vi "Main.vi"(8 "Error In":errorcluster, 11 "Simulate hardware?":bool) -> (0 "Error Out":errorcluster)   [LabVIEW 2017, in "Colour Wheel.lvlib"]
uses:
  Colour Wheel.lvlib
  Controls/Commands [enum].ctl
  Controls/Params.ctl
  Events/Controls/Action Refs [enum].ctl
  <vilib>/Utility/error.llb/Error Cluster From Error Code.vi
  <vilib>/ErrorRing/Error Ring.xnode
  System Control/Main controller.lvlib
  File IO/File IO.lvlib
  Events/Events.lvlib
  Thorlabs_FW102C/Thorlabs_FW102C.lvlib
panel:
  in  "Index":i32=1
  out "Connected?":bool
  out "COM Ports":string[](array[string])
  out "Test":bool=TRUE
  in  "Config":T1
  out "Config out":T1
  in  "Set state":T2
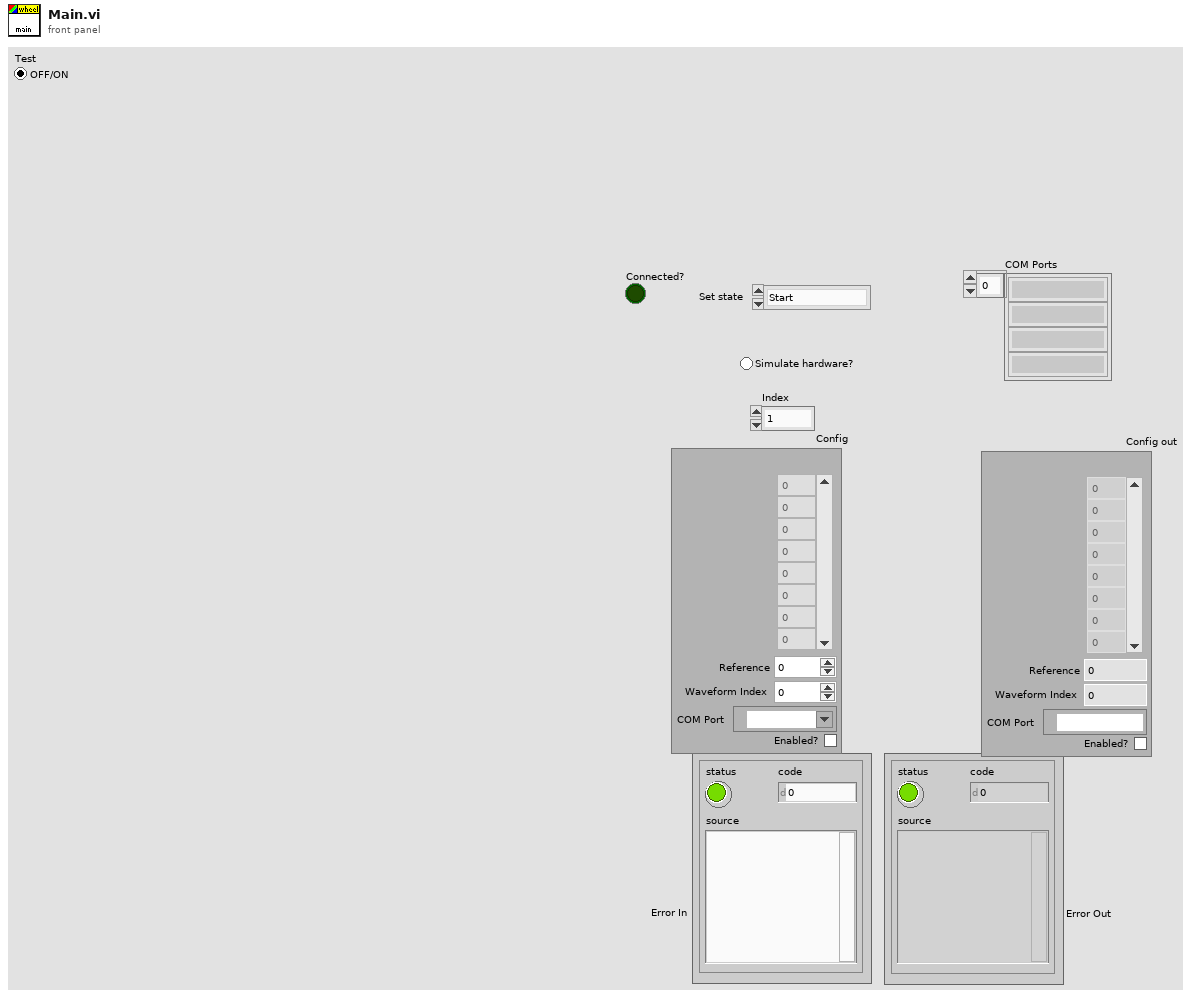
[diagram p1: front panel]
types:
  T1 = typedef "Colour Wheel.lvlib/Params.ctl" = cluster{"Reference":i32, "Colour Wheel Wavelengths":dbl[], "Waveform Index":i32, "COM Port":refnum<visa-resource-name>, "Enabled?":bool}
  T2 = typedef "Colour Wheel.lvlib/Commands [enum].ctl" = enum16{"Start", "Move", "Get position", "Stop", "Send data"}
  T3 = enum32{"Bad", "Idle", "Run top level", "Running"}
  T4 = typedef "Events.lvlib/Action Refs [enum].ctl" = enum16{"Init", "Ref", "Kill"}
  T5 = typedef "Events.lvlib/Refs [cluster].ctl" = cluster{"Exit":refnum<user-event>, "Controller":refnum<user-event>, "System Error":refnum<user-event>, "UI":refnum<user-event>, "Example Module":refnum<user-event>, "Shutter":refnum<user-event>, "Monochromator":refnum<user-event>, "DAQ":refnum<user-event>, "Scope":refnum<user-event>, "Processing":refnum<user-event>, "File IO":refnum<user-event>, "Colour wheel":refnum<user-event>}
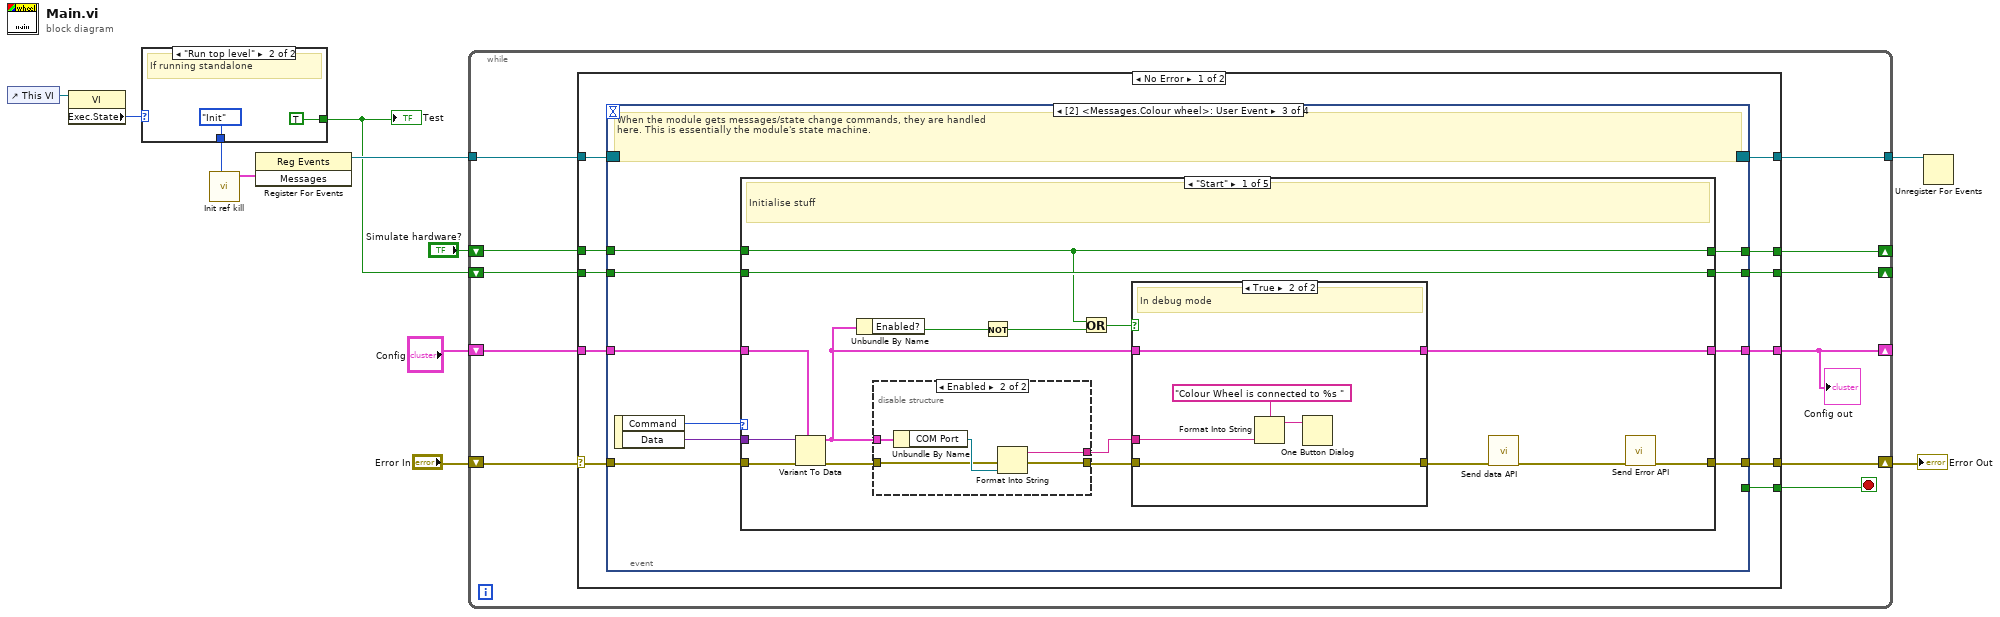
[diagram p0: block diagram]
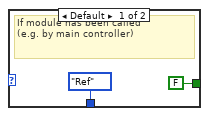
[diagram p2: hidden frame]
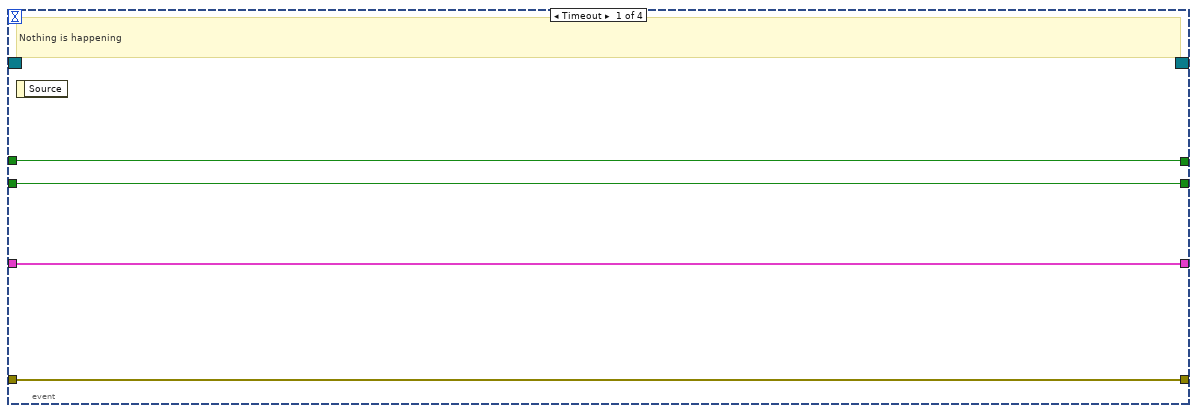
[diagram p3: hidden frame]
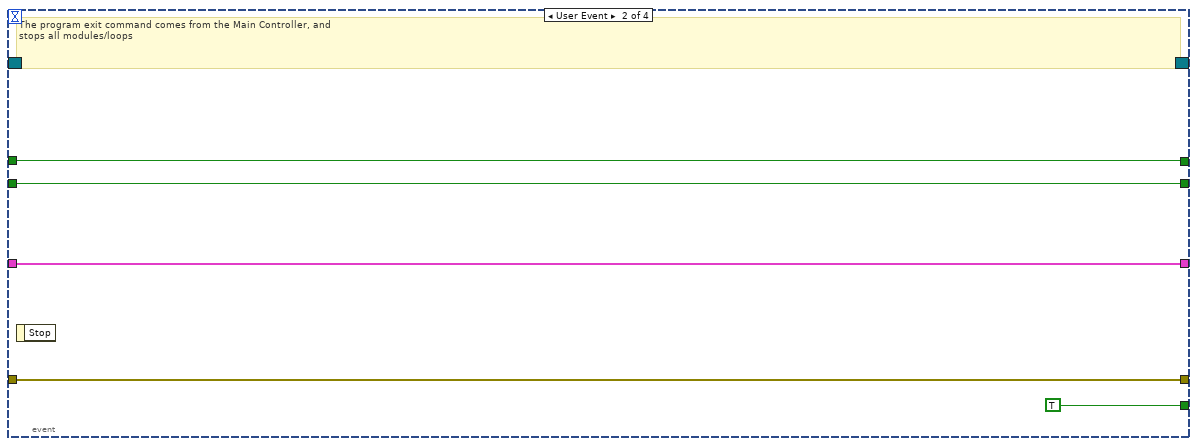
[diagram p4: hidden frame]
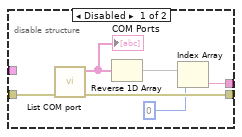
[diagram p5: hidden frame]
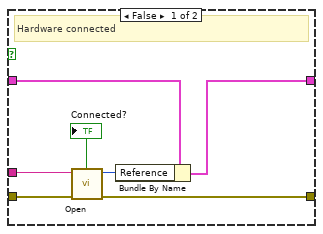
[diagram p6: hidden frame]
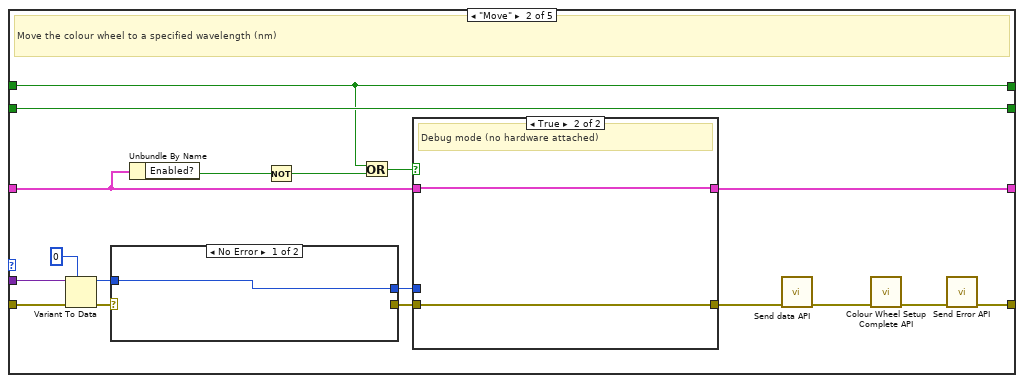
[diagram p7: hidden frame]
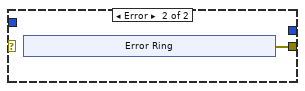
[diagram p8: hidden frame]
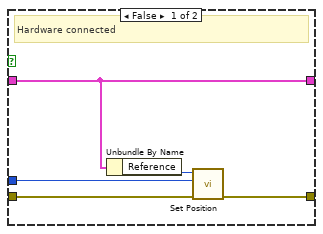
[diagram p9: hidden frame]
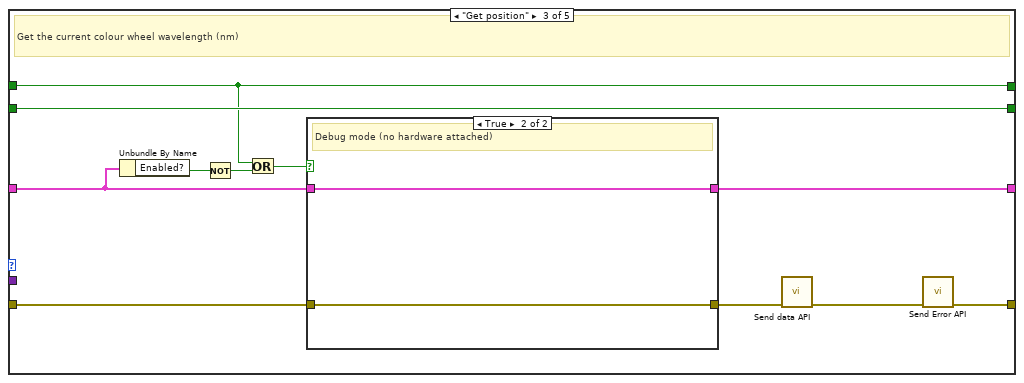
[diagram p10: hidden frame]
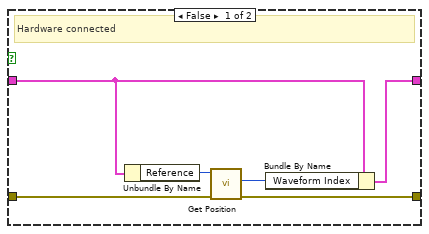
[diagram p11: hidden frame]
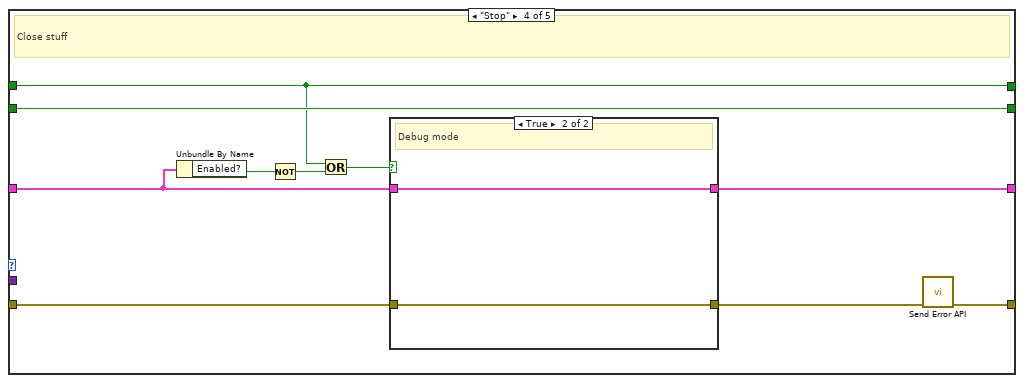
[diagram p12: hidden frame]
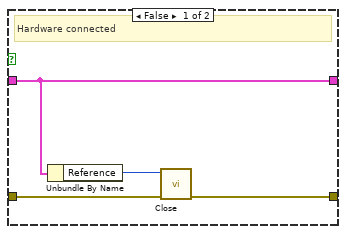
[diagram p13: hidden frame]
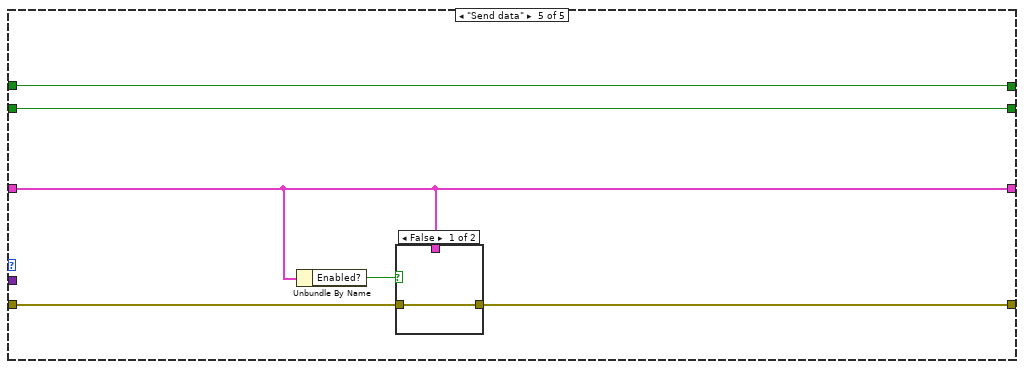
[diagram p14: hidden frame]
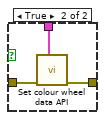
[diagram p15: hidden frame]
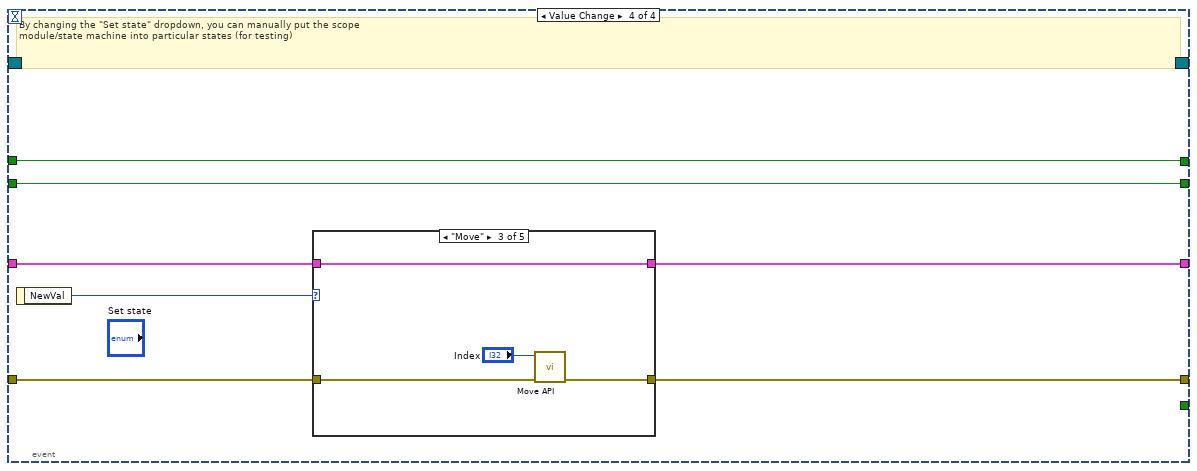
[diagram p16: hidden frame]
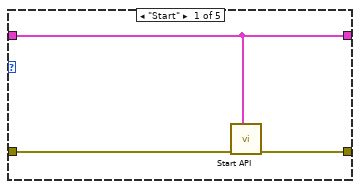
[diagram p17: hidden frame]
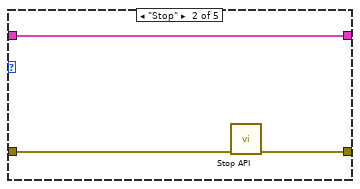
[diagram p18: hidden frame]
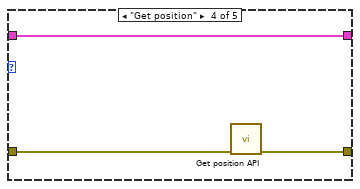
[diagram p19: hidden frame]
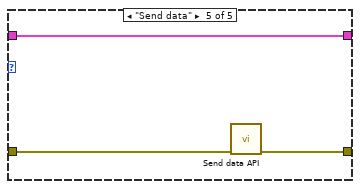
[diagram p20: hidden frame]
diagram:
  n1 = control-ref of="This VI"() -> (w5:refnum<vi>)
  n2 = property class="VI"(reference=w5) -> ("Exec.State"=w4:T3)  [unwired: 1 in, 2 out]
  n3 = case shown="\"Run top level\"" w4 {
    tunnel: [Action_Refs_[enum]."Ref" ("Action") Action_Refs_[enum]."Init" ("Action")] -> w3
    tunnel: [FALSE TRUE] -> w2
    frame Default {
      # "If module has been called\n(e.g. by main controller)"
    }
    frame "Run top level" {
      # "If running standalone"
    }
  }
  "Test" <- w2
  n4 = call "Init ref kill.vi"("Action"=w3) -> ("Messages"=w11:T5)  [unwired: 9 in, 1 out]
  n5 = register-events(w11) -> (reference out=w10:refnum<event-registration>)  [unwired: 2 in, 1 out]
  n6 = while {
    tunnel: w10 -> [w26]
    tunnel: [w24] -> w9
    shift-right: [w21] -> w7
    shift-left: "Error In" -> [w22]
    shift-right: [w16] -> _
    shift-left: "Config" -> [w23]
    shift-right: [w19] -> _
    shift-left: w2 -> [w20]
    shift-right: [w17] -> _
    shift-left: "Simulate hardware?" -> [w18]
    stop <- w25 stop-if-true
    n7 = case shown="No Error" w22 {
      selector: w22 -> [w31 w200]
      tunnel: w26 -> [w37 w198]
      tunnel: [w36 _] -> w25
      tunnel: [w35 w198] -> w24
      tunnel: w23 -> [w34 w199]
      tunnel: [w33 w199] -> w16
      tunnel: [w32 w201] -> w21
      tunnel: w20 -> [w30 w196]
      tunnel: [w29 w196] -> w19
      tunnel: w18 -> [w28 w197]
      tunnel: [w27 w197] -> w17
      frame No Error {
        n8 = event shown="[2] <Messages.Colour wheel>: User Event" {
          selector: w37 -> [_ _ _ _]
          dyn-events: [_ _ _ _] -> w35
          timeout: _ -> [_ _ _ _]
          tunnel: [_ TRUE _ _] -> w36
          tunnel: w31 -> [w41 w45 w48 w177]
          tunnel: [w41 w45 w54 w176] -> w32
          tunnel: w34 -> [w40 w44 w47 w178]
          tunnel: [w40 w44 w53 w175] -> w33
          tunnel: w30 -> [w39 w43 w52 w174]
          tunnel: [w39 w43 w51 w174] -> w29
          tunnel: w28 -> [w38 w42 w50 w173]
          tunnel: [w38 w42 w49 w173] -> w27
          event Timeout {
            # "Nothing is happening"
            n9 = event-data() -> ()  [unwired: 1 in, 1 out]
          }
          event User Event {
            # "The program exit command comes from the Main Controller, and \nstops all modules/loops"
            n10 = event-data() -> ()  [unwired: 1 in, 1 out]
          }
          event User Event {
            # "When the module gets messages/state change commands, they are handled \nhere. This is essentially the module's state machine."
            n11 = event-data() -> ("Command"=w56:T2, "Data"=w55:variant)  [unwired: 1 in]
            n12 = case shown="\"Start\"" w56 {
              tunnel: w55 -> [w70 w109 _ _ _]
              tunnel: w48 -> [w71 w110 w133 w152 w166]
              tunnel: [w72 w113 w137 w156 w165] -> w54
              tunnel: w47 -> [w69 w99 w131 w150 w164]
              tunnel: [w67 w104 w136 w153 w164] -> w53
              tunnel: w52 -> [w65 w111 w134 w155 w168]
              tunnel: [w65 w111 w134 w155 w168] -> w51
              tunnel: [w60 w98 w130 w149 w167] -> w49
              tunnel: w50 -> [w60 w98 w130 w149 w167]
              frame "Start" {
                # "Initialise stuff"
                n13 = Variant To Data(error in=w71, type=w69, Variant=w70) -> (data=w57:T1, error out=w64:errorcluster)
                n14 = Unbundle By Name(w57) -> ("Enabled?"=w61:bool)
                n15 = disable-structure shown="Enabled" {
                  disable-tunnel: w64 -> [w76 w79]
                  disable-tunnel: [w75 w81] -> w63
                  disable-tunnel: [w74 w80] -> w62
                  disable-tunnel: w57 -> [_ w83]
                  frame Disabled {
                    n16 = call "List COM port.vi"("error in (no error)"=w76) -> ("error out"=w74:errorcluster, "COM Ports"=w78:string[])  [unwired: 9 in]
                    "COM Ports" <- w78
                    n17 = Reverse 1D Array(array=w78) -> (reversed array=w77:string[])
                    n18 = Index Array(array=w77, index=0) -> (element=w75:string)
                  }
                  frame Enabled {
                    n19 = Unbundle By Name(w83) -> ("COM Port"=w82:refnum<visa-resource-name>)
                    n20 = Format Into String(error in=w79, w82) -> (resulting string=w81:string, error out=w80:errorcluster)  [unwired: 2 in]
                  }
                }
                n21 = Not(x=w61) -> (.not. x?=w58:bool)
                n22 = Or(x=w60, y=w58) -> (x .or. y?=w59:bool)
                n23 = case shown="True" w59 {
                  tunnel: w57 -> [w85 w95]
                  tunnel: [w86 w95] -> w67
                  tunnel: w62 -> [w89 w94]
                  tunnel: [w88 w94] -> w66
                  tunnel: w63 -> [w90 w91]
                  frame False {
                    # "Hardware connected"
                    n24 = call "Open.vi"("error in (no error)"=w89, "Serial Port"=w90) -> ("error out"=w88:errorcluster, "FW102C out"=w87:i32, "Connected?"=→"Connected?":bool)  [unwired: 7 in]
                    n25 = Bundle By Name(cluster=w85, "Reference"=w87) -> (w86:T1)
                  }
                  frame True {
                    # "In debug mode"
                    n26 = Format Into String(format string="Colour Wheel is connected to %s ", w91) -> (resulting string=w93:string)  [unwired: 2 in, 1 out]
                    n27 = One Button Dialog(message=w93) -> ()  [unwired: 1 in, 1 out]
                  }
                }
                n28 = call "Send data API.vi"("Error In"=w66) -> ("Error Out"=w68:errorcluster)  [unwired: 10 in]
                n29 = call "Send Error API.vi"("Error Cluster"=w68) -> ("Error Out"=w72:errorcluster)  [unwired: 10 in]
              }
              frame "Move" {
                # "Move the colour wheel to a specified wavelength (nm)"
                n30 = Variant To Data(error in=w110, type=0 ("Waveform Index"), Variant=w109) -> (data=w106:i32, error out=w108:errorcluster)
                n31 = case shown="No Error" w108 {
                  tunnel: [_ w115] -> w107
                  tunnel: [w114 _] -> w105
                  tunnel: w106 -> [w114 _]
                  frame No Error {
                  }
                  frame Error {
                    n32 = xnode "Error Ring"() -> ("error out"=w115:errorcluster)
                  }
                }
                n33 = Unbundle By Name(w99) -> ("Enabled?"=w100:bool)
                n34 = Not(x=w100) -> (.not. x?=w96:bool)
                n35 = Or(x=w98, y=w96) -> (x .or. y?=w97:bool)
                n36 = case shown="True" w97 {
                  tunnel: [w124 w126] -> w112
                  tunnel: w107 -> [w125 w126]
                  tunnel: w105 -> [w123 _]
                  tunnel: w99 -> [w121 w127]
                  tunnel: [w121 w127] -> w104
                  frame False {
                    # "Hardware connected"
                    n37 = Unbundle By Name(w121) -> ("Reference"=w122:i32)
                    n38 = call "Set Position.vi"("error in (no error)"=w125, "Index"=w123, "FW102C in"=w122) -> ("error out"=w124:errorcluster)  [unwired: 7 in, 1 out]
                  }
                  frame True {
                    # "Debug mode (no hardware attached)"
                  }
                }
                n39 = call "Send data API.vi"("Error In"=w112) -> ("Error Out"=w103:errorcluster)  [unwired: 10 in]
                n40 = call "Colour Wheel Setup Complete API.vi"("Error In"=w103) -> ("Error Out"=w102:errorcluster)  [unwired: 10 in]
                n41 = call "Send Error API.vi"("Error Cluster"=w102) -> ("Error Out"=w113:errorcluster)  [unwired: 10 in]
              }
              frame "Get position" {
                # "Get the current colour wheel wavelength (nm)"
                n42 = Unbundle By Name(w131) -> ("Enabled?"=w132:bool)
                n43 = Not(x=w132) -> (.not. x?=w128:bool)
                n44 = Or(x=w130, y=w128) -> (x .or. y?=w129:bool)
                n45 = case shown="True" w129 {
                  tunnel: w131 -> [w141 w146]
                  tunnel: [w140 w146] -> w136
                  tunnel: [w143 w145] -> w135
                  tunnel: w133 -> [w144 w145]
                  frame False {
                    # "Hardware connected"
                    n46 = Unbundle By Name(w141) -> ("Reference"=w142:i32)
                    n47 = call "Get Position.vi"("error in (no error)"=w144, "FW102C in"=w142) -> ("error out"=w143:errorcluster, "Position"=w139:i32)  [unwired: 7 in, 1 out]
                    n48 = Bundle By Name(cluster=w141, "Waveform Index"=w139) -> (w140:T1)
                  }
                  frame True {
                    # "Debug mode (no hardware attached)"
                  }
                }
                n49 = call "Send data API.vi"("Error In"=w135) -> ("Error Out"=w138:errorcluster)  [unwired: 10 in]
                n50 = call "Send Error API.vi"("Error Cluster"=w138) -> ("Error Out"=w137:errorcluster)  [unwired: 10 in]
              }
              frame "Stop" {
                # "Close stuff"
                n51 = Unbundle By Name(w150) -> ("Enabled?"=w151:bool)
                n52 = Not(x=w151) -> (.not. x?=w147:bool)
                n53 = Or(x=w149, y=w147) -> (x .or. y?=w148:bool)
                n54 = case shown="True" w148 {
                  tunnel: [w160 w162] -> w154
                  tunnel: [w159 w161] -> w153
                  tunnel: w150 -> [w159 w161]
                  tunnel: w152 -> [w157 w162]
                  frame False {
                    # "Hardware connected"
                    n55 = Unbundle By Name(w159) -> ("Reference"=w158:i32)
                    n56 = call "Close.vi"("error in (no error)"=w157, "FW102C in"=w158) -> ("error out"=w160:errorcluster)  [unwired: 9 in]
                  }
                  frame True {
                    # "Debug mode"
                  }
                }
                n57 = call "Send Error API.vi"("Error Cluster"=w154) -> ("Error Out"=w156:errorcluster)  [unwired: 10 in]
              }
              frame "Send data" {
                n58 = Unbundle By Name(w164) -> ("Enabled?"=w163:bool)
                n59 = case shown="False" w163 {
                  tunnel: w166 -> [w169 w172]
                  tunnel: [w169 w171] -> w165
                  tunnel: w164 -> [_ w170]
                  frame False {
                  }
                  frame True {
                    n60 = call "Set colour wheel data API.vi"("Colour wheel"=w170, "Error In"=w172) -> ("Error Out"=w171:errorcluster)  [unwired: 9 in]
                  }
                }
              }
            }
          }
          event Value Change {
            # "By changing the \"Set state\" dropdown, you can manually put the scope \nmodule/state machine into particular states (for testing)"
            n61 = event-data() -> ("NewVal"=w179:T2)  [unwired: 1 in]
            n62 = case shown="\"Move\"" w179 {
              tunnel: w178 -> [w180 w185 w189 w192 w195]
              tunnel: [w180 w185 w189 w192 w195] -> w175
              tunnel: [w181 w183 w187 w190 w193] -> w176
              tunnel: w177 -> [w182 w184 w188 w191 w194]
              frame "Start" {
                n63 = call "Start API.vi"("Colour wheel"=w180, "Error In"=w182) -> ("Error Out"=w181:errorcluster)  [unwired: 9 in]
              }
              frame "Stop" {
                n64 = call "Stop API.vi"("Error In"=w184) -> ("Error Out"=w183:errorcluster)  [unwired: 10 in]
              }
              frame "Move" {
                n65 = call "Move API.vi"("Error In"=w188, "Index"="Index") -> ("Error Out"=w187:errorcluster)  [unwired: 9 in]
              }
              frame "Get position" {
                n66 = call "Get position API.vi"("Error In"=w191) -> ("Error Out"=w190:errorcluster)  [unwired: 10 in]
              }
              frame "Send data" {
                n67 = call "Send data API.vi"("Error In"=w194) -> ("Error Out"=w193:errorcluster)  [unwired: 10 in]
              }
            }
          }
        }
      }
      frame Error {
        n68 = case shown="False" w196 {
          tunnel: [w203 _] -> w201
          tunnel: w200 -> [w202 w207]
          frame False {
            n69 = case shown="Error" w202 {
              selector: w202 -> [w204 w205]
              tunnel: [w204 w206] -> w203
              frame No Error {
              }
              frame Error {
                n70 = call "Log error API.vi"("Error In"=w205) -> ("Error Out"=w206:errorcluster)  [unwired: 10 in]
              }
            }
          }
          frame True {
            n71 = call <vilib>:"Simple Error Handler.vi"("error in (no error)"=w207) -> ()  [unwired: 4 in, 5 out]
          }
        }
      }
    }
    "Config out" <- w16
  }
  "Error Out" <- w7
  n72 = Unregister For Events(event registration refnum=w9) -> ()  [unwired: 1 in, 1 out]
